vi "RSZVB Set Sweep Segment Triggering.vi"(7 "Triggering (On)":bool=TRUE, 8 "error in (no error)":errorcluster {"code" format="%.0x"}, 9 "Segment (1)":i32=1, 10 "Channel (1)":i32=1, 11 "VISA resource name":refnum<visa-resource-name>) -> (0 "error out":errorcluster {"code" format="%.0x"}, 3 "VISA resource name out":refnum<visa-resource-name>)   [LabVIEW 2011]
doc: "This VI deactivates/activates triggering for segment <Seg>. This setting only takes effect if:\n\n1. The analyzer is not in Free Run mode (see rszvb_SetTriggerSource)\n\n2. Selective segment triggering is enabled (RSZVB Set Sweep Selective Segment Triggering.vi set to ON) \n\nRemote-control command(s):\n[SENSe<Ch>:]SEGMent<Seg>:TRIGger:STATe"
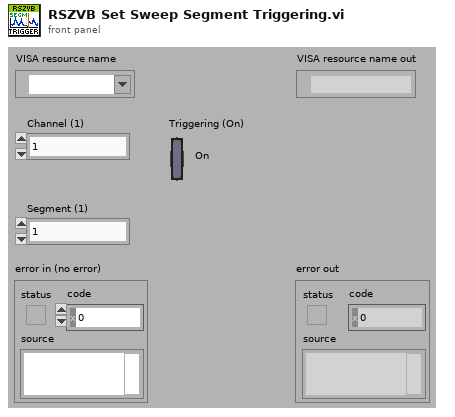
[diagram p1: front panel]
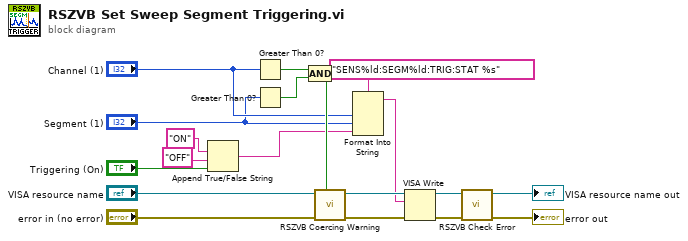
[diagram p0: block diagram]
diagram:
  n1 = Append True/False String(1:"Triggering (On)", 2:"OFF", 3:"ON") -> (0:w10:string)  [unwired: 1 in]
  n2 = Greater Than 0?(x="Channel (1)") -> (x > 0?=w9:bool)
  n3 = Greater Than 0?(x="Segment (1)") -> (x > 0?=w8:bool)
  n4 = Compound Arithmetic op=AND(w9, w8) -> (w14:bool)
  n5 = call "RSZVB Coercing Warning.vi"("In Range?"=w14, "error in (no error)"="error in (no error)", "VISA session"="VISA resource name") -> ("error out"=w17:errorcluster, "dup VISA session"=w18:refnum<visa-resource-name>)  [unwired: 7 in]
  n6 = Format Into String(format string="SENS%ld:SEGM%ld:TRIG:STAT %s", "Channel (1)", "Segment (1)", w10) -> (resulting string=w13:string)  [unwired: 2 in, 1 out]
  n7 = VISA Write(VISA resource name=w18, write buffer=w13, error in (no error)=w17) -> (VISA resource name out=w15:refnum<visa-resource-name>, error out=w16:errorcluster)  [unwired: 1 out]
  n8 = call "RSZVB Check Error.vi"("error in (no error)"=w16, "VISA session"=w15) -> ("error out"=→"error out":errorcluster, "dup VISA session"=→"VISA resource name out":refnum<visa-resource-name>)  [unwired: 8 in]
